vi "DataTransmissionTcpWriter.vi"() -> ()   [LabVIEW 2009]
uses:
  Data Transmission/TransmissionState.ctl
  lib/Data Access Objects/Metadata/Persistant DAO Actions.ctl
  lib/Launcher/Launcher Actions.ctl
  lib/Launcher/NoPanelAppTypes.ctl
  lib/Apps/App Status Actions.ctl
panel:
  in  "Save":bool
  in  "Port Number":u16=6445
  out "Transmission State":T1=enum."Transmitting"
  out "Sending Data":bool
  in  "Wait For Notification Timeout":i32=1000000
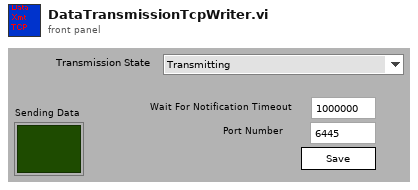
[diagram p1: front panel]
types:
  T1 = typedef "TransmissionState.ctl" = enum16{"Listening", "Transmitting", "Disconnecting"}
  T2 = typedef "Persistant DAO Actions.ctl" = enum16{"Init", "Get", "Set", "Load", "Save"}
  T3 = typedef "NoPanelAppTypes.ctl" = enum16{"NTCP Socket", "Data Archiving", "DAQ Link", "Control Loops", "Autobalance Monitor", "Mixed Mode Monitor", "Cart Plot", "Act Plot", "Cmd Disp Diffs"}
  T4 = typedef "Launcher Actions.ctl" = enum16{"Launch", "Stop All", "Stop", "Kill", "Running?", "Init"}
  T5 = typedef "Network Parameters.ctl" = cluster{"Port Number In":u16, "Notification Name In":string, "Wait For Notification Timeout In":i32}
  T6 = typedef "App Status Actions.ctl" = enum16{"Init", "Get Status", "Running", "Control", "Autobalanced", "Data Acquisition", "Set App State", "DAQ Started", "Set LBCB State", "Set All", "Set Cont Logging", "Set Step Logging", "Set MM Logging", "Set Volt Logging", "Set Cart Type", "Set DAQ Link", "Set NTCP Link"}
  T7 = typedef "LBCB Location.ctl" = enum16{"Crane Bay Two LBCB", "Crane Bay One LBCB", "5th Scale Two LBCB", "5th Scale One LBCB", "Portable LBCB"}
  T8 = typedef "App Status.ctl" = cluster{"Running":bool, "Controlling L2":bool, "Autobalance L2":bool, "Data Acquisition":bool, " App State":T9, "DAQ Started":bool, "LBCB 1 State":T10, "LBCB 2 State":T10, "Controlling L1":bool, "Autobalance L1":bool, "Cartesian Type":bool, "Continuous Logging":bool, "Step Logging":bool, "Voltage Logging":bool, "Mixed Mode Logging":bool, "DAQ Link":bool, "NTCP Link ":bool}
  T9 = typedef "AppStates.ctl" = enum16{"Starting OM", "Initializing Displays", "Setting up Archiving", "Setting Up DAQ Channels", "Start DAQ", "DAQ Starting", "Controlling LBCBs", "Stopping OM"}
  T10 = typedef "Lbcb Control Loop States.ctl" = enum16{"Idle", "Start Selected", "Load Last Command", "Start Autobalancing", "Autobalancing", "Control Loop Initialized", "Control Enabled"}
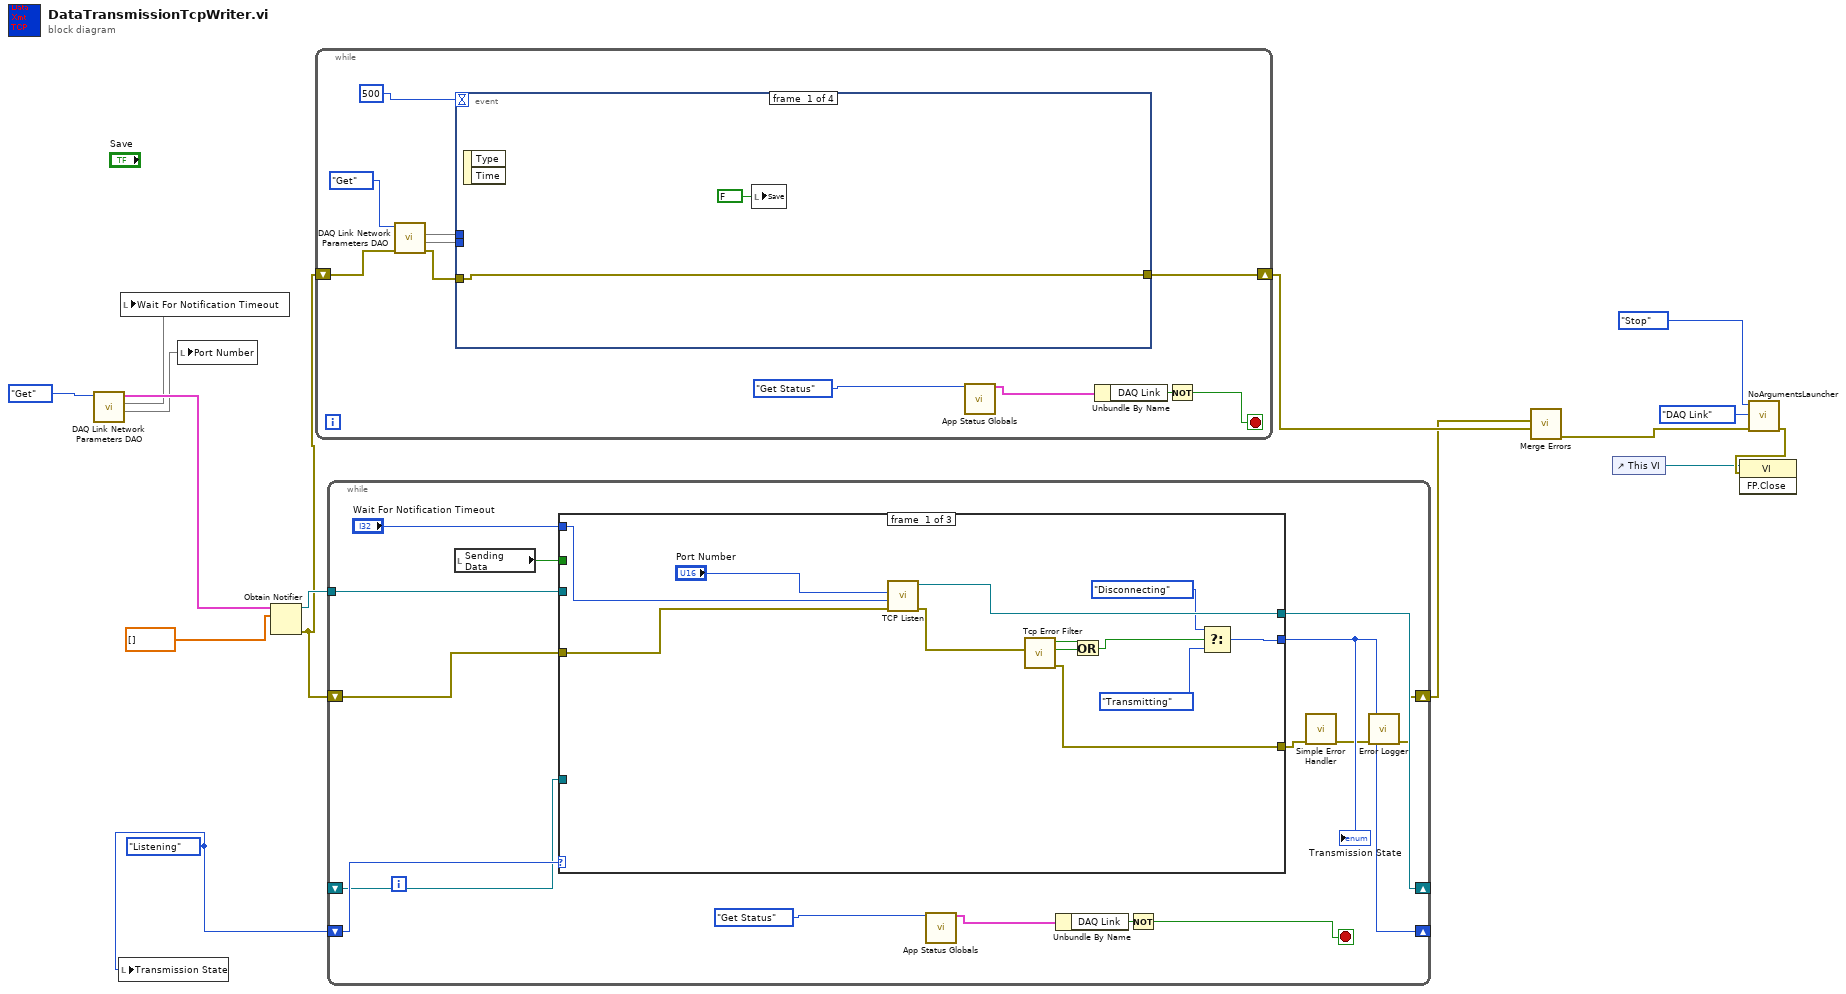
[diagram p0: block diagram]
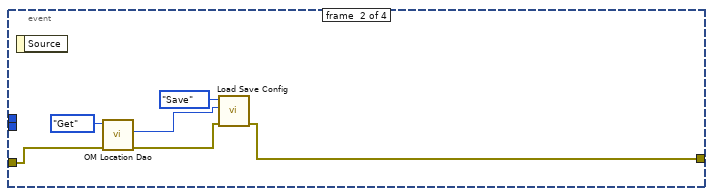
[diagram p2: hidden frame]
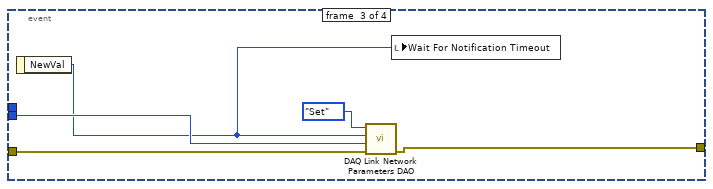
[diagram p3: hidden frame]
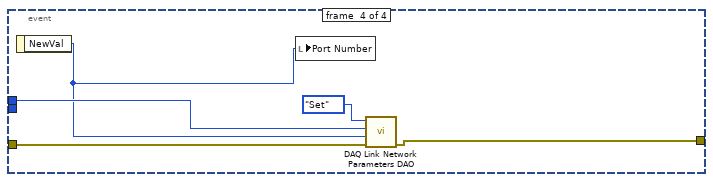
[diagram p4: hidden frame]
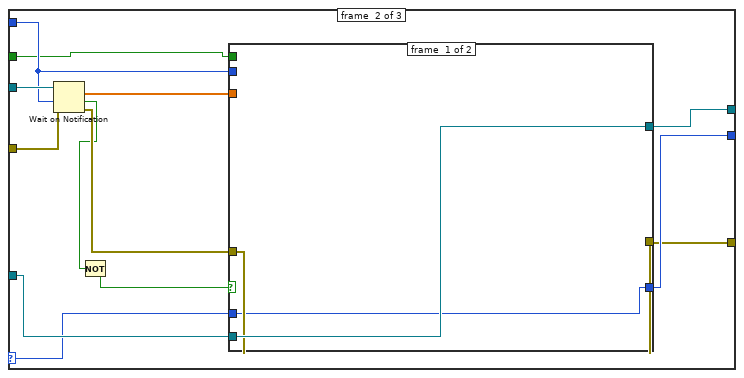
[diagram p5: hidden frame]
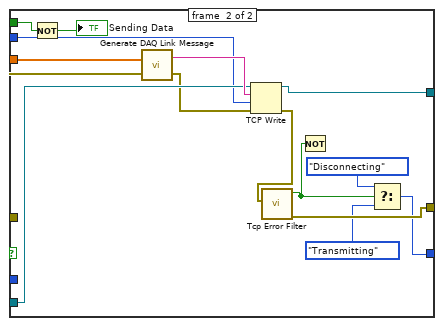
[diagram p6: hidden frame]
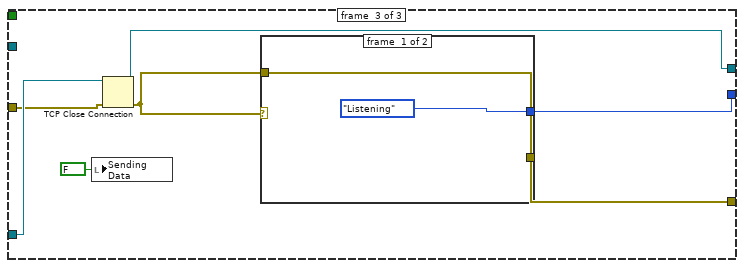
[diagram p7: hidden frame]
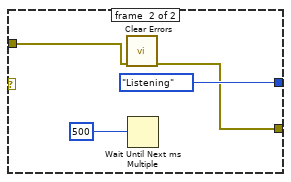
[diagram p8: hidden frame]
diagram:
  w14 = TransmissionState."Listening" ("Transmission State 2")
  n1 = call "DAQ Link Network Parameters DAO.vi"("Persistent DAO Actions"=Persistant_DAO_Actions."Get") -> (1:w1, 2:w2, "Network Parameters Out"=w12:T5)  [unwired: 2 in, 6 out]
  n2 = local write "Transmission State"(w14) -> ()
  n3 = local write "Wait For Notification Timeout"(w2) -> ()
  n4 = local write "Port Number"(w1) -> ()
  n5 = Obtain Notifier(name (unnamed)=w12, notification data type=dbl[] [] ("appended array")) -> (notifier out=w15:refnum<notifier>, error out=w4:errorcluster)  [unwired: 2 in, 1 out]
  n6 = while {
    shift-right: [w22] -> w7
    shift-left: w4 -> [w24]
    stop <- w17 stop-if-true
    n7 = call "DAQ Link Network Parameters DAO.vi"("error in (no error)"=w24, "Persistent DAO Actions"=Persistant_DAO_Actions."Get") -> ("error out"=w23:errorcluster, 1:w25, 2:w26)  [unwired: 1 in, 6 out]
    n8 = event shown="[1] \"Save\": Mouse Down" {
      selector: _ -> [_ _ _ _]
      dyn-events: _ -> [_ _ _ _]
      timeout: 500 -> [_ _ _ _]
      tunnel: w26 -> [_ _ _ w41]
      tunnel: w25 -> [_ _ w39 _]
      tunnel: w23 -> [w28 w32 w38 w44]
      tunnel: [w28 w33 w37 w43] -> w22
      event #0 {
        n9 = event-data() -> ()  [unwired: 3 out]
        n10 = local write "Save"(FALSE ("Save")) -> ()
      }
      event #1 {
        n11 = event-data() -> ()  [unwired: 2 out]
        n12 = call "OM Location Dao.vi"("error in (no error)"=w32, "Actions"=Persistant_DAO_Actions."Get") -> ("error out"=w31:errorcluster, "LBCB  Location Out"=w30:T7)  [unwired: 2 in, 6 out]
        n13 = call "Load Save Config.vi"("error in (no error)"=w31, "OM  Location"=w30, "Actions"=Persistant_DAO_Actions."Save") -> ("error out"=w33:errorcluster)  [unwired: 8 out]
      }
      event #2 {
        n14 = event-data() -> ("NewVal"=w35:i32)  [unwired: 1 out]
        n15 = call "DAQ Link Network Parameters DAO.vi"("error in (no error)"=w38, 9:w39, 10:w35, "Persistent DAO Actions"=Persistant_DAO_Actions."Set") -> ("error out"=w37:errorcluster)  [unwired: 1 in, 6 out]
        n16 = local write "Wait For Notification Timeout"(w35) -> ()
      }
      event #3 {
        n17 = event-data() -> ("NewVal"=w40:u16)  [unwired: 1 out]
        n18 = local write "Port Number"(w40) -> ()
        n19 = call "DAQ Link Network Parameters DAO.vi"("error in (no error)"=w44, 9:w40, 10:w41, "Persistent DAO Actions"=Persistant_DAO_Actions."Set") -> ("error out"=w43:errorcluster)  [unwired: 1 in, 6 out]
      }
    }
    n20 = call "App Status Globals.vi"("App Status Actions"=App_Status_Actions."Get Status") -> ("App Status Out"=w19:T8)  [unwired: 5 in, 9 out]
    n21 = Unbundle By Name(w19) -> ("DAQ Link"=w18:bool)
    n22 = Not(x=w18) -> (.not. x?=w17:bool)
  }
  n23 = while {
    shift-right: [w59] -> _
    shift-left: _ -> [w56]
    shift-right: [w51] -> w5
    shift-left: w4 -> [w58]
    shift-right: [w54] -> _
    shift-left: w14 -> [w57]
    tunnel: w15 -> [w55]
    stop <- w46 stop-if-true
    n24 = local read "Sending Data"() -> (w45:bool)
    n25 = case shown="\"Transmitting\"" w57 {
      selector: w57 -> [_ w74 _]
      tunnel: [w71 w80 w108] -> w59
      tunnel: w58 -> [w70 w83 w107]
      tunnel: [w61 w75 w104] -> w52
      tunnel: [w62 w76 w106] -> w54
      tunnel: w56 -> [_ w81 w109]
      tunnel: w55 -> [_ w84 _]
      tunnel: "Wait For Notification Timeout" -> [w69 w73 _]
      tunnel: w45 -> [_ w72 _]
      frame #0 {
        n26 = call <vilib>:"TCP Listen.vi"("error in (no error)"=w70, "timeout ms (wait forever: -1)"=w69, "port"="Port Number") -> ("error out"=w68:errorcluster, "connection ID"=w71:refnum<k5>)  [unwired: 1 in, 6 out]
        n27 = call "Tcp Error Filter.vi"("error in (no error)"=w68) -> ("error out"=w61:errorcluster, "Timed Out"=w66:bool, "Lost"=w67:bool)  [unwired: 8 out]
        n28 = Or(x=w67, y=w66) -> (x .or. y?=w65:bool)
        n29 = Select(t=TransmissionState."Disconnecting" ("Transmission State 2"), s=w65, f=TransmissionState."Transmitting" ("Transmission State 2")) -> (s? t:f=w62:T1)
      }
      frame #1 {
        n30 = Wait on Notification(notifier=w84, timeout in ms (-1)=w73, error in (no error)=w83) -> (notification=w82:dbl[], timed out?=w78:bool, error out=w79:errorcluster)  [unwired: 2 out]
        n31 = Not(x=w78) -> (.not. x?=w77:bool)
        n32 = case shown="True" w77 {
          tunnel: w82 -> [_ w98]
          tunnel: w81 -> [w87 w101]
          tunnel: [w87 w100] -> w80
          tunnel: w79 -> [w86 w99]
          tunnel: [w86 w94] -> w75
          tunnel: w73 -> [_ w96]
          tunnel: [w85 w90] -> w76
          tunnel: w74 -> [w85 _]
          tunnel: w72 -> [_ w88]
          frame #0 {
          }
          frame #1 {
            n33 = Not(x=w88) -> (.not. x?=→"Sending Data":bool)
            n34 = call "Generate DAQ Link Message.vi"("error in"=w99, "All Data"=w98) -> ("error out"=w97:errorcluster, "Message"=w102:string)
            n35 = TCP Write(connection ID=w101, data in=w102, error in (no error)=w97, 9:w96) -> (connection ID out=w100:refnum<k5>, error out=w95:errorcluster)  [unwired: 1 out]
            n36 = call "Tcp Error Filter.vi"("error in (no error)"=w95) -> ("error out"=w94:errorcluster, "Lost"=w92:bool)  [unwired: 9 out]
            n37 = Not(x=w92) -> ()  [unwired: 1 out]
            n38 = Select(t=TransmissionState."Disconnecting" ("Transmission State 2"), s=w92, f=TransmissionState."Transmitting" ("Transmission State 2")) -> (s? t:f=w90:T1)
          }
        }
      }
      frame #2 {
        n39 = local write "Sending Data"(FALSE ("Sending Data")) -> ()
        n40 = TCP Close Connection(connection ID=w109, error in (no error)=w107) -> (connection ID out=w108:refnum<k5>, error out=w105:errorcluster)  [unwired: 1 out]
        n41 = case shown="Error" w105 {
          tunnel: [TransmissionState."Listening" ("Transmission State 2") TransmissionState."Listening" ("Transmission State 2")] -> w106
          tunnel: w105 -> [w110 w113]
          tunnel: [w110 w112] -> w104
          frame #0 {
          }
          frame #1 {
            n42 = call <vilib>:"Clear Errors.vi"("error in (no error)"=w113) -> ("error out"=w112:errorcluster)  [unwired: 6 out]
            n43 = Wait Until Next ms Multiple(millisecond multiple=500) -> ()  [unwired: 1 out]
          }
        }
      }
    }
    "Transmission State" <- w54
    n44 = call "App Status Globals.vi"("App Status Actions"=App_Status_Actions."Get Status") -> ("App Status Out"=w48:T8)  [unwired: 5 in, 9 out]
    n45 = Unbundle By Name(w48) -> ("DAQ Link"=w47:bool)
    n46 = Not(x=w47) -> (.not. x?=w46:bool)
    n47 = call <vilib>:"Simple Error Handler.vi"("error in (no error)"=w52) -> ("error out"=w50:errorcluster)  [unwired: 1 in, 7 out]
    n48 = call "Error Logger.vi"("error in (no error)"=w50) -> ("error out"=w51:errorcluster)  [unwired: 1 in, 9 out]
  }
  n49 = call <vilib>:"Merge Errors.vi"("error in 3 (no error)"=w7, "error in 2 (no error)"=w5) -> ("error out"=w6:errorcluster)  [unwired: 2 in, 3 out]
  n50 = control-ref of="This VI"() -> (w10:refnum<vi>)
  n51 = call "NoArgumentsLauncher.vi"("error in (no error)"=w6, "Application"=NoPanelAppTypes."DAQ Link", "Application Launcher Actions"=Launcher_Actions."Stop") -> ("error out"=w11:errorcluster)  [unwired: 8 out]
  n52 = invoke class="VI" method="FP.Close"(reference=w10, error in=w11) -> ()  [unwired: 1 in, 3 out]
